vi "measure_rpm_winAvg.vi"() -> ()   [LabVIEW 2019]
uses:
  <vilib>/myRIO/Common/Instrument Driver Framework/myRIO v1.0/IRQ/typedefs/DI IRQ Type.ctl
  <vilib>/userDefined/High Color/nirio_resource_hc.ctl
  <vilib>/Platform/TimedLoop/XDataNode/timing_clust.ctl
  <vilib>/Platform/TimedLoop/XDataNode/nitl_modes.ctl
  <vilib>/Platform/TimedLoop/XDataNode/wakeup.ctl
  rpm.vi
  ISR.vi
  <vilib>/myRIO/Common/Instrument Driver Framework/myRIO v1.0/IRQ/vis/myRIO v1.1 Register DI IRQ.vi
  <vilib>/myRIO/Common/Instrument Driver Framework/myRIO v1.0/IRQ/vis/myRIO v1.0 Reserve IRQ.vi
  <vilib>/myRIO/Common/Instrument Driver Framework/Utilities/vis/FPGA Ref Manager.vi
  <vilib>/myRIO/Common/Instrument Driver Framework/myRIO v1.0/myRIO v1.0 Close.vi
  <vilib>/Utility/file.llb/Write Delimited Spreadsheet (DBL).vi
  <vilib>/myRIO/Express VI/IRQ/IRQ Express VI.xnode
  <vilib>/myRIO/Instrument Drivers/IRQ/IO IRQ/vis/myRIO Register DI IRQ.xnode
  <vilib>/myRIO/Common/Instrument Driver Framework/myRIO v1.0/IRQ/typedefs/Callback VI Ref.ctl
  <vilib>/platform/TimedLoop/XDataNode/XDataNode.xnode
  <vilib>/Platform/TimedLoop/XDataNode/XDNodeRunTimeDep.lvlib
  <vilib>/myRIO/Instrument Drivers/IRQ/IO IRQ/IO IRQ.lvlib
panel:
  out "N":i32
  out "Final i":i32
  out "Error":errorcluster
  out "Max. Iteration Duration":i64
  out "error out (no error) 2":errorcluster
  in  "RPM Inst Data":path=path "/tmp/log.csv"
  out "Omega":dbl[](graph)
  out "Iteration Duration":i64
  out "Finished late":bool
  out "Interrupt On":bool
  in  "error in (no error)":errorcluster
  out "Np":dbl
  out "ft":dbl
  out "omega_vec":dbl[](array[numeric])
  out "k_p":dbl
  out "g_p":dbl
  in  "Run Time (s)":dbl
  in  "Sampling \nFrequency (Hz)":dbl
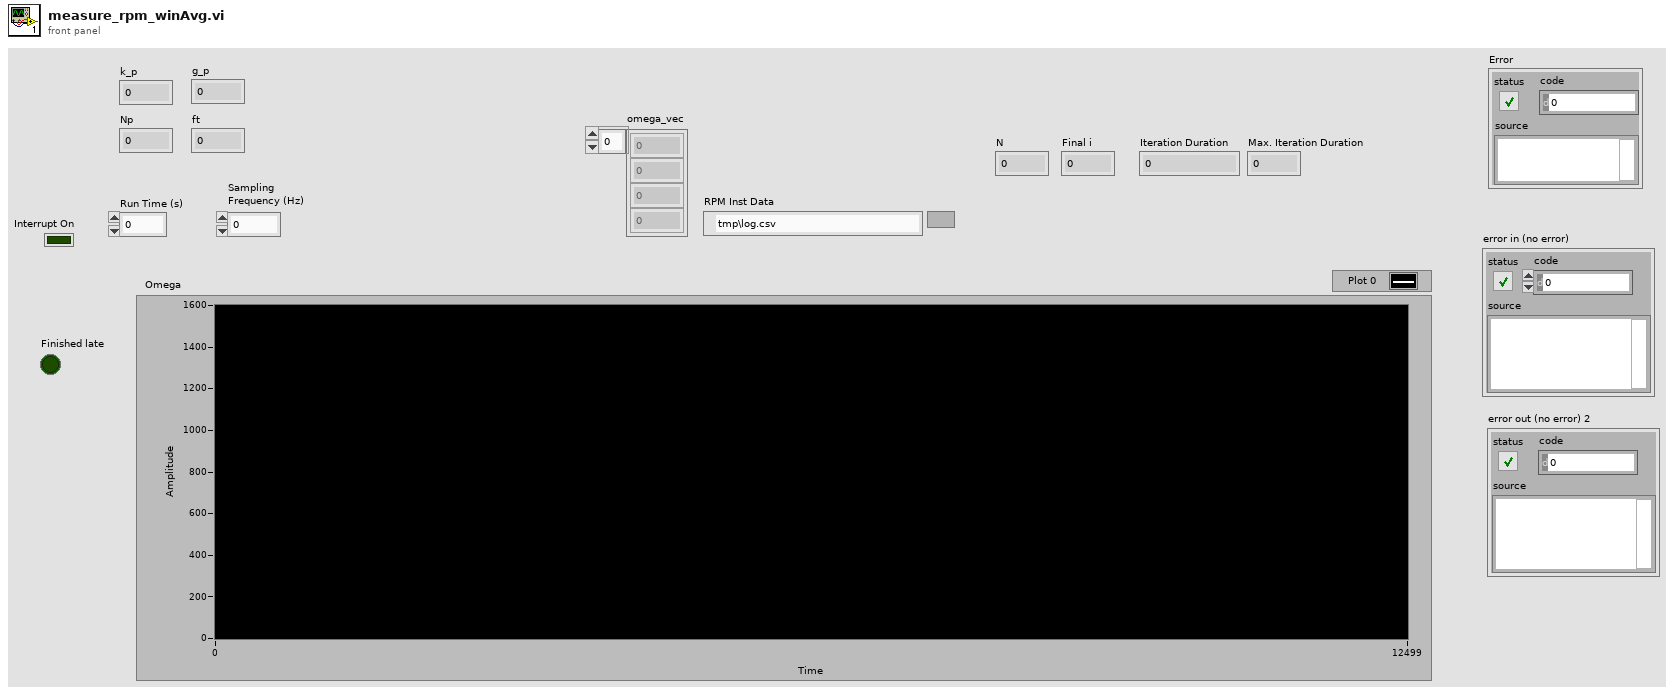
[diagram p1: front panel]
types:
  T1 = typedef "XDNodeRunTimeDep.lvlib/timing_clust.ctl" = cluster{"Expected End [f-1]":u64, "Actual End [f-1]":u64, "Finished Late? [f-1]":bool, "Expected End [i-1]":u64, "Actual End [i-1]":u64, "Finished Late? [i-1]":bool, "Expected Start [i]":u64, "Actual Start [i]":u64, "Expected Start [f]":u64, "Actual Start [f]":u64, "Source Name":string, "Structure Name":string, "Period":i64, "Deadline":i64, "Offset":i64, "Start":i64, "Priority":i32, "Timeout":i32, "Mode":T2, "Wakeup Reason":T3, "Error":errorcluster, "Source Type":string, "Secondary Source Type":string, "Global End Time":u64, "Global Start Time":u64, "Frame Duration":u64, "Iteration Duration":u64, "Assigned CPU":i32, "I/O Scan Engine Mode":u32}
  T2 = typedef "XDNodeRunTimeDep.lvlib/nitl_modes.ctl" = enum32{"No Change", "Process missed periods, maintain original phase", "Discard missed periods, maintain original phase", "Process missed periods, ignore original phase", "Discard missed periods, ignore original phase"}
  T3 = typedef "XDNodeRunTimeDep.lvlib/wakeup.ctl" = enum32{"Normal", "Aborted", "Asynchronous wakeup", "Timing source error", "Timed loop error", "Timeout"}
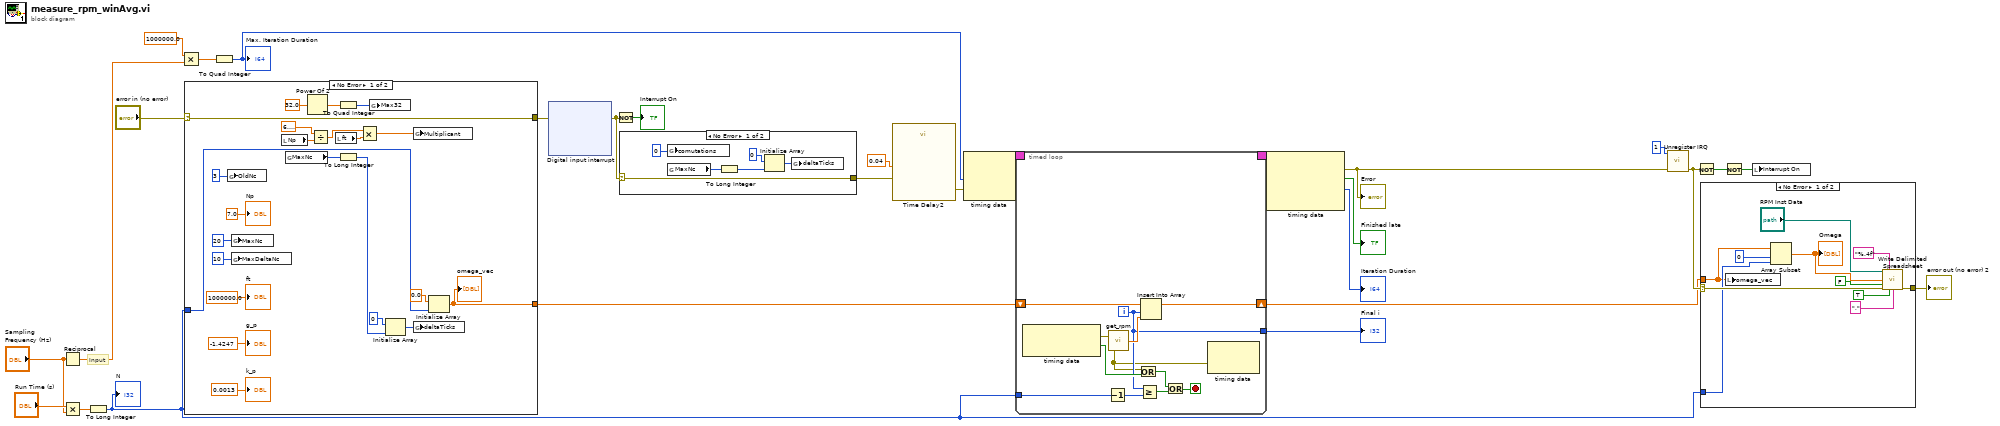
[diagram p0: block diagram]
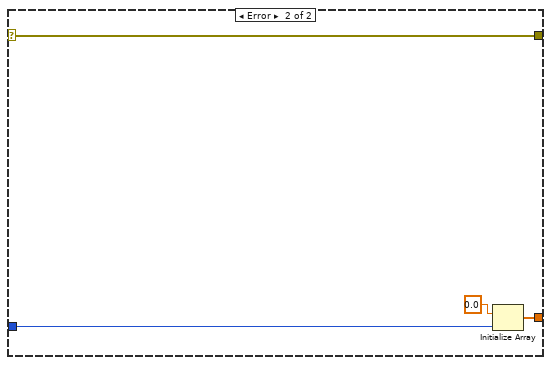
[diagram p4: hidden frame]
diagram:
  # "Input"
  n1 = Reciprocal(x="Sampling \nFrequency (Hz)") -> (1/x=w13:dbl)
  n2 = Multiply(x="Run Time (s)", y="Sampling \nFrequency (Hz)") -> (x*y=w26:dbl)
  n3 = To Long Integer(number=w26) -> (32bit integer=w6:i32)
  "N" <- w6
  n4 = Multiply(x=1000000.0, y=w13) -> (x*y=w16:dbl)
  n5 = case shown="No Error" "error in (no error)" {
    selector: "error in (no error)" -> [w48 w55]
    tunnel: [w48 w55] -> w21
    tunnel: w6 -> [w36 w52]
    tunnel: [w29 w53] -> w3
    frame No Error {
      n6 = global write "rpm.vi" "OldNc"(i64 3 ("MaxNc")) -> ()
      n7 = global write "rpm.vi" "MaxNc"(i64 20 ("MaxNc")) -> ()
      n8 = global write "rpm.vi" "MaxDeltaNc"(i64 10 ("MaxDeltaNc")) -> ()
      n9 = local read "Np"() -> (w44:dbl)
      n10 = global read "rpm.vi" "MaxNc"() -> (w33:i64)
      n11 = Power Of 2(x=32.0) -> (2^x=w50:dbl)
      n12 = Divide(x=6.283185307179586, y=w44) -> (x/y=w43:dbl)
      n13 = local read "ft"() -> (w42:dbl)
      n14 = To Quad Integer(1:w50) -> (0:w41:i64)
      n15 = To Long Integer(number=w33) -> (32bit integer=w32:i32)
      n16 = Multiply(x=w43, y=w42) -> (x*y=w51:dbl)
      n17 = global write "rpm.vi" "Max32"(w41) -> ()
      n18 = Initialize Array(i64 0, w32) -> (w34:i64[])
      n19 = global write "rpm.vi" "Multiplicant"(w51) -> ()
      n20 = global write "rpm.vi" "deltaTicks"(w34) -> ()
      n21 = Initialize Array(0.0 ("element"), w36) -> (w29:dbl[])
      "omega_vec" <- w29
      "Np" <- 7.0 ("Numeric")
      "ft" <- 1000000.0 ("ft")
      "k_p" <- 0.0013 ("k_p")
      "g_p" <- -1.4247 ("g_p")
    }
    frame Error {
      n22 = Initialize Array(0.0 ("element"), w52) -> (w53:dbl[])
    }
  }
  n23 = To Quad Integer(1:w16) -> (0:w15:i64)
  "Max. Iteration Duration" <- w15
  n24 = xnode "Digital input interrupt"("error in (no error)"=w21) -> ("error out"=w2:errorcluster)
  n25 = Not(x=w2) -> (.not. x?=→"Interrupt On":bool)
  n26 = case shown="No Error" w2 {
    selector: w2 -> [w60 w62]
    tunnel: [w60 w62] -> w19
    frame No Error {
      n27 = global write "rpm.vi" "comutations"(i64 0 ("comutations")) -> ()
      n28 = global read "rpm.vi" "MaxNc"() -> (w57:i64)
      n29 = To Long Integer(number=w57) -> (32bit integer=w56:i32)
      n30 = Initialize Array(i64 0, w56) -> (w58:i64[])
      n31 = global write "rpm.vi" "deltaTicks"(w58) -> ()
    }
    frame Error {
    }
  }
  n32 = call "Time Delay2"("error in (no error)"=w19, "Delay Time (s)"=0.04) -> ("error out"=w24:errorcluster)  [unwired: 9 in]
  n33 = node-c288(w15, w24) -> (w28:T1)  [unwired: 1 in]
  n34 = timed-loop {
    timing: w28 -> [_]
    timing-out: [_] -> w27
    tunnel: w6 -> [w66]
    shift-right: [w67] -> w5
    shift-left: w3 -> [w68]
    tunnel: [w64] -> w4
    i -> [w64]
    stop <- w74 stop-if-true
    n35 = node-c288() -> (w71:errorcluster, w69:bool)  [unwired: 1 in]
    n36 = Decrement(x=w66) -> (x-1=w65:i32)
    n37 = call "get_rpm.vi"("error in (no error)"=w71) -> ("RPM"=w70:dbl, "error out"=w63:errorcluster)
    n38 = Or(x=w63, y=w69) -> (x .or. y?=w73:bool)
    n39 = Greater Or Equal?(x=w64, y=w65) -> (x >= y?=w72:bool)
    n40 = Insert Into Array(array=w68, index=w64, new element=w70) -> (w67:dbl[])
    n41 = Or(x=w73, y=w72) -> (x .or. y?=w74:bool)
    n42 = node-c288(w63) -> ()  [unwired: 1 in, 1 out]
  }
  "Final i" <- w4
  n43 = node-c288(w27) -> (w1:errorcluster, →"Finished late":bool, →"Iteration Duration":i64)  [unwired: 1 out]
  "Error" <- w1
  n44 = call <vilib>:"Unregister IRQ.vi"("error in (no error)"=w1, "IRQ Number"=u8 1) -> ("error out"=w8:errorcluster)  [unwired: 9 in]
  n45 = Not(x=w8) -> (.not. x?=w12:bool)
  n46 = case shown="No Error" w8 {
    selector: w8 -> [w86 w92]
    tunnel: [w85 w92] -> w7
    tunnel: w6 -> [w82 _]
    tunnel: w5 -> [w81 _]
    frame No Error {
      n47 = local write "omega_vec"(w81) -> ()
      n48 = Array Subset(array=w81, index=0, length=w82) -> (w84:dbl[])
      "Omega" <- w84
      n49 = call-poly <vilib>:"Write Delimited Spreadsheet.vi"("file path (dialog if empty)"="RPM Inst Data", "format (%.3f)"="%.4f", "1D data"=w84, "append to file? (new file:F)"=FALSE, "error in (no error)"=w86, "transpose? (no:F)"=TRUE, "delimiter (\\t)"="," ("delimiter (\\t)")) -> ("error out"=w85:errorcluster)  [unwired: 7 in, 1 out]
    }
    frame Error {
    }
  }
  "error out (no error) 2" <- w7
  n50 = Not(x=w12) -> (.not. x?=w11:bool)
  n51 = local write "Interrupt On"(w11) -> ()
